vi "Map Source to Dest.vi"(8 "error in (no error)":errorcluster, 10 "Source":i32, 11 "Map in":refnum<class "Map.lvclass">) -> (0 "error out":errorcluster, 2 "Destination":i32, 3 "Map out":refnum<class "Map.lvclass">)   [LabVIEW 2020, in "Map.lvclass"]
uses:
  Map.lvclass
  Map.lvclass/Map.ctl
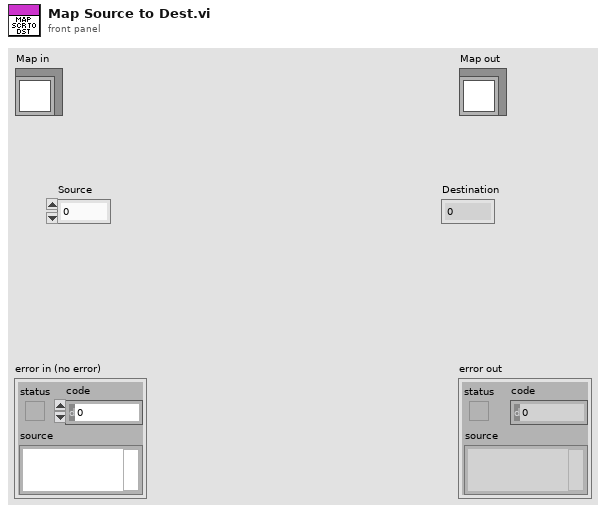
[diagram p1: front panel]
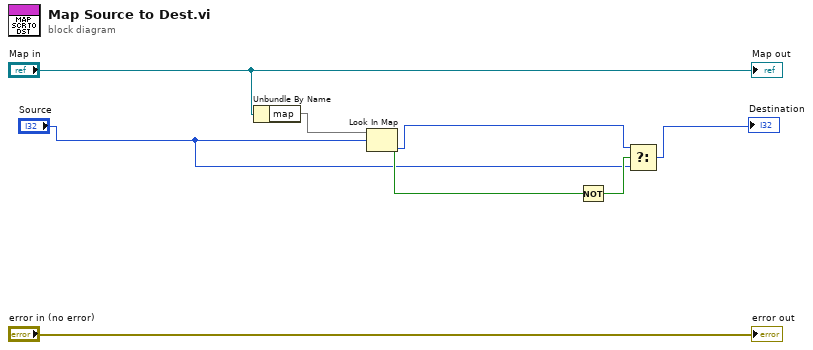
[diagram p0: block diagram]
diagram:
  n1 = Unbundle By Name("Map in") -> ("map"=w6:map{i32, i32})
  n2 = Look In Map(map=w6, key="Source") -> (key not found?=w5:bool, value=w2:i32)  [unwired: 1 in]
  n3 = Not(x=w5) -> (.not. x?=w4:bool)
  n4 = Select(t=w2, s=w4, f="Source") -> (s? t:f=→"Destination":i32)
  "error out" <- "error in (no error)"
  "Map out" <- "Map in"
